vi "HCalFile.vi"   [LabVIEW 2009]
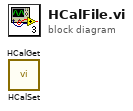
[diagram p0: block diagram]
diagram:
  n1 = call "HCalSet.vi"() -> ()  [unwired: 2 in, 1 out]
  n2 = call "HCalGet.vi"() -> ()  [unwired: 2 in, 1 out]
